vi "find_common_bboxes.vi"(0 "Scores L":dbl[](array[numeric]), 1 "Class nums L":dbl[](array[numeric]), 5 "BBoxes L":dbl[][](array[numeric]), 7 "Class nums R":dbl[](array[numeric]), 9 "Scores R":dbl[](array[numeric]), 11 "error in (no error)":errorcluster, 12 "BBoxes R":dbl[][](array[numeric])) -> (4 "Common classes":dbl[](array[numeric]), 6 "Common bboxes [y, x]":dbl[][](array[numeric]), 8 "Scores L":dbl[](array[numeric]), 10 "Scores R":dbl[](array[numeric]), 15 "error out":errorcluster)   [LabVIEW 2019]
uses:
  57e90a8b-a7b6-49be-a029-412614f4c8cb.vi
  acb91e0a-be20-4d63-8254-3041dc949d50.vi
  8fe12e6d-21d4-479d-8595-ea26008ef021.vi
  9c4d7369-aa4b-4996-98af-ade1cf9e3b87.vi
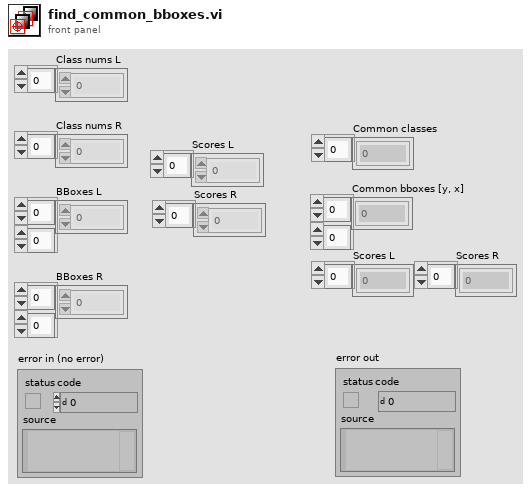
[diagram p1: front panel]
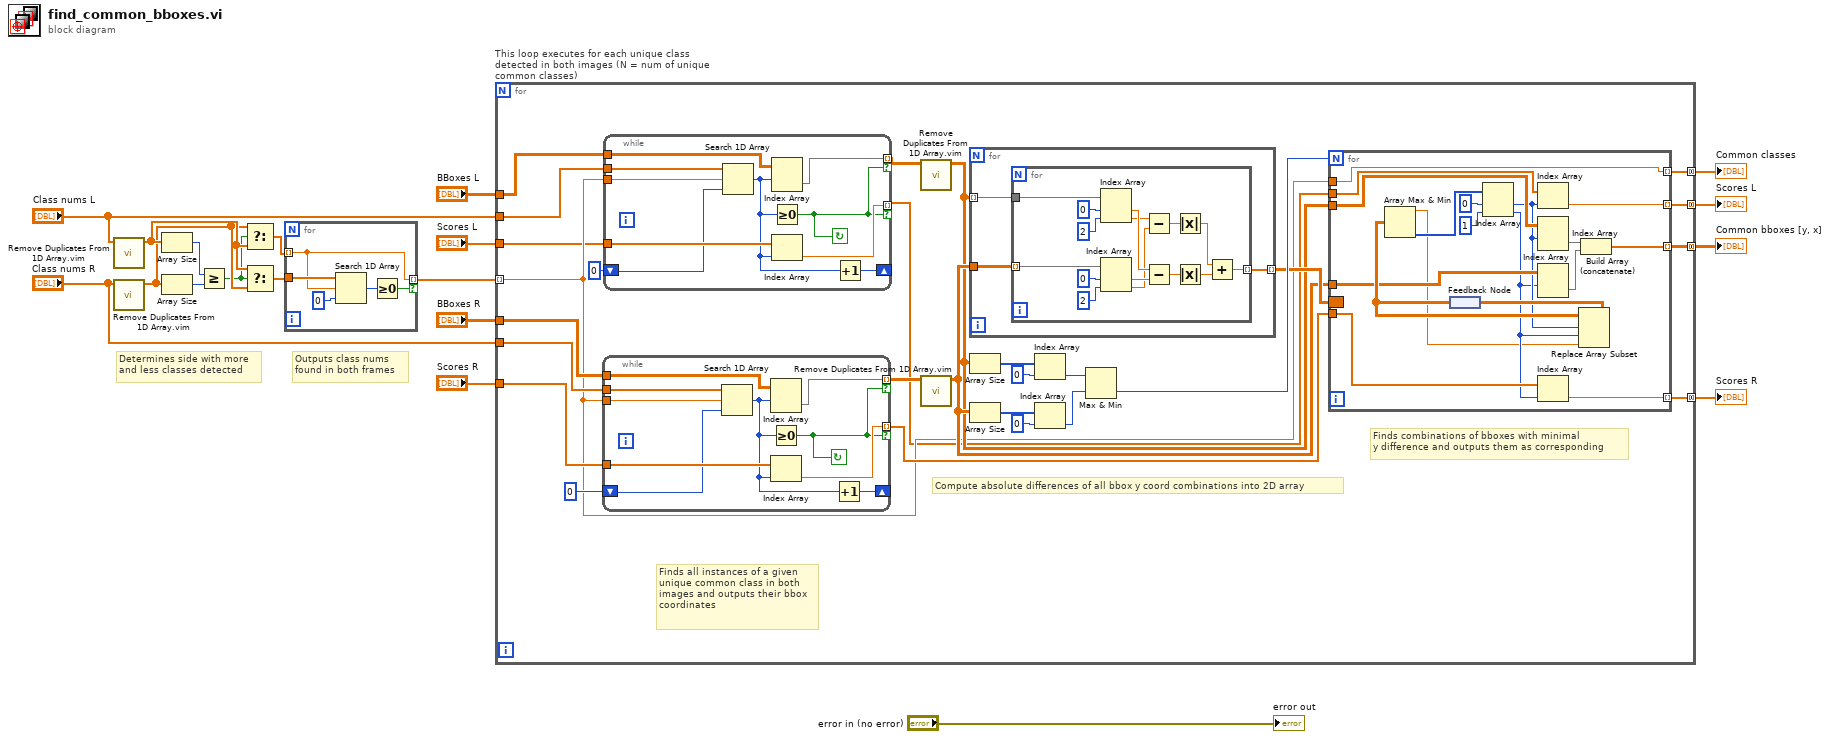
[diagram p0: block diagram]
diagram:
  # "Outputs class nums \nfound in both frames"
  # "Determines side with more\nand less classes detected"
  n1 = call "Remove Duplicates From 1D Array.vim"("array"="Class nums L") -> ("array with duplicates removed"=w14:dbl[])  [unwired: 10 in]
  n2 = call "Remove Duplicates From 1D Array.vim"("array"="Class nums R") -> ("array with duplicates removed"=w11:dbl[])  [unwired: 10 in]
  n3 = Array Size(array=w14) -> (size(s)=w9:i32)
  n4 = Array Size(array=w11) -> (size(s)=w8:i32)
  n5 = Greater Or Equal?(x=w9, y=w8) -> (x >= y?=w10:bool)
  n6 = Select(t=w11, s=w10, f=w14) -> (s? t:f=w12:dbl[])
  n7 = Select(t=w14, s=w10, f=w11) -> (s? t:f=w13:dbl[])
  n8 = for {
    tunnel: w12 -> [w20] mode=indexing
    tunnel: w13 -> [w24]
    tunnel: [w20] -> w15 mode=indexing if=w21
    n9 = Search 1D Array(1D array=w24, element=w20, start index (0)=0) -> (index of element=w22:i32)
    n10 = Greater Or Equal To 0?(x=w22) -> (x >= 0?=w21:bool)
  }
  n11 = for "This loop executes for each unique class detected in both images (N = num of unique common classes)" {
    tunnel: w15 -> [w29] mode=indexing
    tunnel: "Class nums L" -> [w30]
    tunnel: "Class nums R" -> [w51]
    tunnel: "BBoxes L" -> [w31]
    tunnel: "BBoxes R" -> [w50]
    tunnel: [w42] -> w2 mode=concatenating
    tunnel: [w37] -> w7 mode=concatenating
    tunnel: "Scores L" -> [w28]
    tunnel: "Scores R" -> [w36]
    tunnel: [w34] -> w4 mode=concatenating
    tunnel: [w33] -> w3 mode=concatenating
    # "Finds combinations of bboxes with minimal \ny difference and outputs them as corresponding"
    # "Compute absolute differences of all bbox y coord combinations into 2D array"
    # "Finds all instances of a given unique common class in both images and outputs their bbox coordinates"
    n12 = while {
      tunnel: w51 -> [w106]
      tunnel: w29 -> [w107]
      tunnel: [w105] -> w40 mode=indexing if=w101
      tunnel: w50 -> [w104]
      tunnel: w36 -> [w103]
      tunnel: [w102] -> w35 mode=indexing if=w101
      shift-right: [w99] -> _
      shift-left: 0 -> [w100]
      stop <- w101 continue-if-true
      n13 = Search 1D Array(1D array=w106, element=w107, start index (0)=w100) -> (index of element=w98:i32)
      n14 = Index Array(array=w104, index (row)=w98) -> (element=w105:dbl[])  [unwired: 1 in]
      n15 = Greater Or Equal To 0?(x=w98) -> (x >= 0?=w101:bool)
      n16 = Index Array(array=w103, index=w98) -> (element=w102:dbl)
      n17 = Increment(x=w98) -> (x+1=w99:i32)
    }
    n18 = while {
      tunnel: w30 -> [w60]
      tunnel: w29 -> [w61]
      tunnel: [w59] -> w26 mode=indexing if=w55
      tunnel: w31 -> [w58]
      tunnel: w28 -> [w57]
      tunnel: [w56] -> w25 mode=indexing if=w55
      shift-right: [w53] -> _
      shift-left: 0 -> [w54]
      stop <- w55 continue-if-true
      n19 = Search 1D Array(1D array=w60, element=w61, start index (0)=w54) -> (index of element=w52:i32)
      n20 = Index Array(array=w58, index (row)=w52) -> (element=w59:dbl[])  [unwired: 1 in]
      n21 = Greater Or Equal To 0?(x=w52) -> (x >= 0?=w55:bool)
      n22 = Index Array(array=w57, index=w52) -> (element=w56:dbl)
      n23 = Increment(x=w52) -> (x+1=w53:i32)
    }
    n24 = call "Remove Duplicates From 1D Array.vim"("array"=w26) -> ("array with duplicates removed"=w38:dbl[][])  [unwired: 10 in]
    n25 = call "Remove Duplicates From 1D Array.vim"("array"=w40) -> ("array with duplicates removed"=w39:dbl[][])  [unwired: 10 in]
    n26 = for "Compute SAD of all bbox y coord combinations" {
      tunnel: w38 -> [w82] mode=indexing
      tunnel: w39 -> [w81]
      tunnel: [w80] -> w41 mode=indexing
      n27 = for {
        tunnel: w82 -> [w97]
        tunnel: w81 -> [w96] mode=indexing
        tunnel: [w83] -> w80 mode=indexing
        n28 = Index Array(array=w97, index #1=0 ("index"), index #2=2 ("index")) -> (element #1=w91:dbl, element #2=w88:dbl)
        n29 = Index Array(array=w96, index #1=0 ("index"), index #2=2 ("index")) -> (element #1=w90:dbl, element #2=w87:dbl)
        n30 = Subtract(x=w88, y=w87) -> (x-y=w86:dbl)
        n31 = Subtract(x=w91, y=w90) -> (x-y=w89:dbl)
        n32 = Absolute Value(x=w86) -> (abs(x)=w85:dbl)
        n33 = Absolute Value(x=w89) -> (abs(x)=w84:dbl)
        n34 = Add(x=w85, y=w84) -> (x+y=w83:dbl)
      }
    }
    n35 = Array Size(array=w38) -> (size(s)=w49:i32[])
    n36 = Array Size(array=w39) -> (size(s)=w48:i32[])
    n37 = Index Array(array=w49, index=0) -> (element=w45:i32)
    n38 = Index Array(array=w48, index=0) -> (element=w44:i32)
    n39 = Max & Min(x=w45, y=w44) -> (min(x,y)=w43:i32)  [unwired: 1 out]
    n40 = for "Finds combinations of bboxes with minimal y difference and outputs them as corresponding" {
      N: w43 -> [_]
      tunnel: w38 -> [w74]
      tunnel: w39 -> [w73]
      border: w41 -> [_]
      tunnel: [w70] -> w42 mode=indexing
      tunnel: w29 -> [w69]
      tunnel: [w69] -> w37 mode=indexing
      tunnel: w25 -> [w68]
      tunnel: w35 -> [w67]
      tunnel: [w64] -> w34 mode=indexing
      tunnel: [w63] -> w33 mode=indexing
      n41 = feedback #1() -> (w78:dbl[][])
      n42 = Array Max & Min(array=w78) -> (max value=w62:dbl, min index (indices)=w77:i32[])  [unwired: 2 out]
      n43 = Index Array(array=w77, index #1=0 ("index"), index #2=1 ("index")) -> (element #1=w66:i32, element #2=w65:i32)
      n44 = Index Array(array=w68, index=w66) -> (element=w64:dbl)
      n45 = Index Array(array=w74, index (row)=w66) -> (element=w72:dbl[])  [unwired: 1 in]
      n46 = Index Array(array=w73, index (row)=w65) -> (element=w71:dbl[])  [unwired: 1 in]
      n47 = Index Array(array=w67, index=w65) -> (element=w63:dbl)
      n48 = Replace Array Subset(array=w78, new element=w62, index (row)=w66, index (col)=w65) -> (w79:dbl[][])
      n49 = feedback-in #1(w79) -> ()
      n50 = Build Array (concatenate)(w72, w71) -> (w70:dbl[])
    }
  }
  "Common bboxes [y, x]" <- w2
  "Common classes" <- w7
  "Scores L" <- w4
  "Scores R" <- w3
  "error out" <- "error in (no error)"
